vi "Error Message.vi"(8 "error in (no error)":errorcluster {"code" format="%.0x"}, 10 "Error Code":i32 format="%.0g", 11 "instrument handle":refnum<k15>) -> (0 "error out":errorcluster {"code" format="%.0x"}, 2 "Error Message":string, 3 "instrument handle out":refnum<k15>)   [LabVIEW 2020, in "Keysight DAQ970.lvlib"]
doc: "Translates the error return value from an IVI driver VI to a user-readable string. The user should pass a buffer with at least 256 bytes for the ErrorMessage parameter."
uses:
  Keysight DAQ970.lvlib
  KtDAQ970.dll
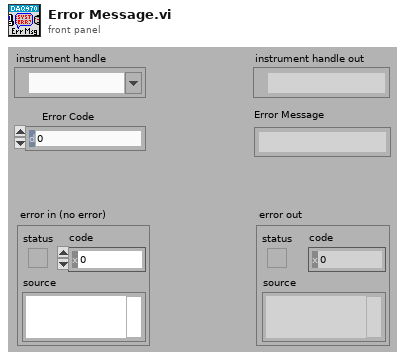
[diagram p1: front panel]
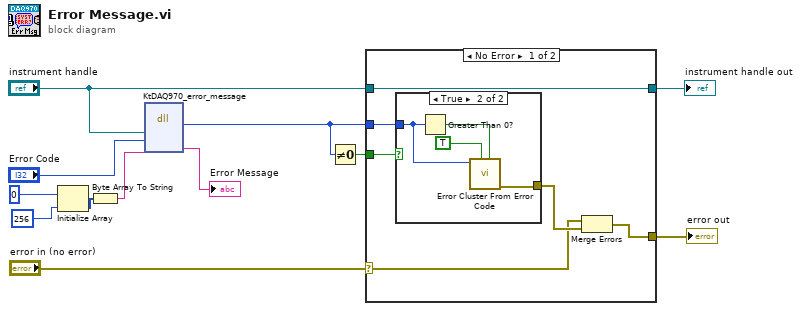
[diagram p0: block diagram]
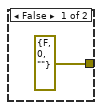
[diagram p2: hidden frame]
diagram:
  n1 = Initialize Array(u8 0, 256) -> (w7:u8[])
  n2 = Byte Array To String(unsigned byte array=w7) -> (string=w10:string)
  n3 = dll-call lib="KtDAQ970**.dll" fn="KtDAQ970_error_message" label="error_message"("instrument handle", "Error Code", w10) -> (w5:i32, →"Error Message":string)  [unwired: 4 in, 3 out]
  n4 = Not Equal To 0?(x=w5) -> (x != 0?=w6:bool)
  n5 = case shown="No Error" "error in (no error)" {
    selector: "error in (no error)" -> [w14 w24]
    tunnel: [w15 w24] -> w4
    tunnel: w6 -> [w18 _]
    tunnel: w5 -> [w17 _]
    tunnel: "instrument handle" -> [w13 w25]
    tunnel: [w13 w25] -> w1
    frame No Error {
      n6 = case shown="True" w18 {
        tunnel: w17 -> [_ w21]
        tunnel: [errorcluster {"status"=FALSE, "code"=0, "source"=""} ("error out") w20] -> w16
        frame False {
        }
        frame True {
          n7 = Greater Than 0?(x=w21) -> (x > 0?=w22:bool)
          n8 = call <vilib>:"Error Cluster From Error Code.vi"("is warning? (False)"=w22, "show call chain? (False)"=TRUE, "error code (0)"=w21) -> ("error out"=w20:errorcluster)  [unwired: 1 in, 5 out]
        }
      }
      n9 = Merge Errors(w14, w16) -> (w15:errorcluster)
    }
    frame Error {
    }
  }
  "instrument handle out" <- w1
  "error out" <- w4
